vi "GT Set Laser Dis Table1D.vi"(0 "cardNum":i16, 1 "minPower":dbl, 2 "pLimitPower":dbl, 5 "count":i16, 7 "pRatio":dbl, 9 "pPos":i32, 11 "error in (no error)":errorcluster caption="错误输入（无错误）", 12 "maxPower":dbl, 13 "channel":i16) -> (4 "pLimitPower out":dbl, 6 "function return":i16, 8 "pRatio out":dbl, 10 "pPos out":i32, 15 "error out":errorcluster caption="错误输出")   [LabVIEW 2014, in "gts.lvlib"]
doc: "GT_API GT_SetLaserDisTable1D(short cardNum,short count,double *pRatio,long *pPos,double minPower,double maxPower,double *pLimitPower,short channel=0);"
uses:
  gts.lvlib
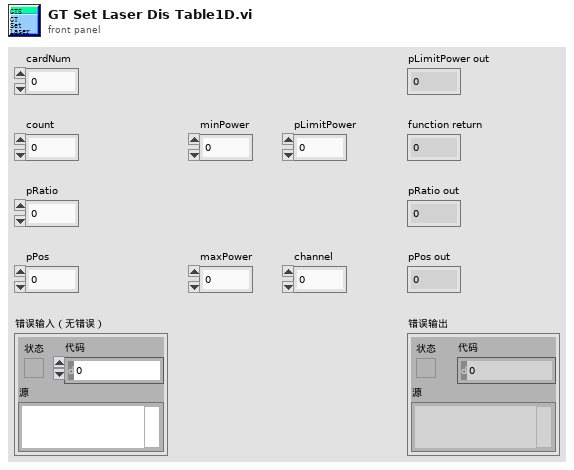
[diagram p1: front panel]
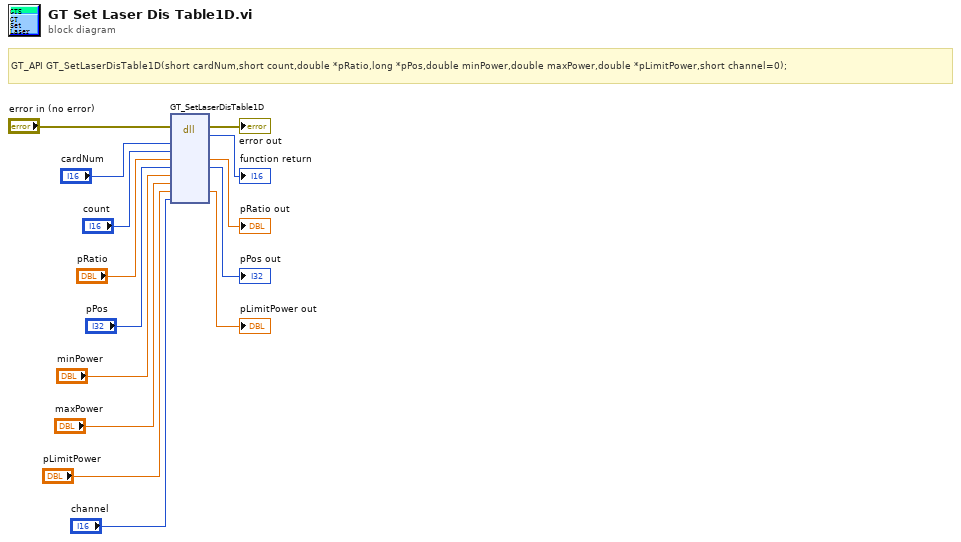
[diagram p0: block diagram]
diagram:
  # "GT_API GT_SetLaserDisTable1D(short cardNum,short count,double *pRatio,long *pPos,double minPower,double maxPower,double *pLimitPower,short channel=0);"
  n1 = dll-call lib="PTH2habs D固高科技资料GTS控制卡GTS卡18年上半年资料dllVC32bit\nmulti_cardgts.*" fn="GT_SetLaserDisTable1D"(error in="error in (no error)", "cardNum"="cardNum", "count"="count", "pRatio"="pRatio", "pPos"="pPos", "minPower"="minPower", "maxPower"="maxPower", "pLimitPower"="pLimitPower", "channel"="channel") -> (error out=→"error out":errorcluster, →"function return":i16, "pRatio"=→"pRatio out":dbl, "pPos"=→"pPos out":i32, "pLimitPower"=→"pLimitPower out":dbl)  [unwired: 7 in, 1 out]
